vi "VENDING MACHINE.vi"() -> ()   [LabVIEW 2019]
panel:
  out "appended array":T1(array[cluster])
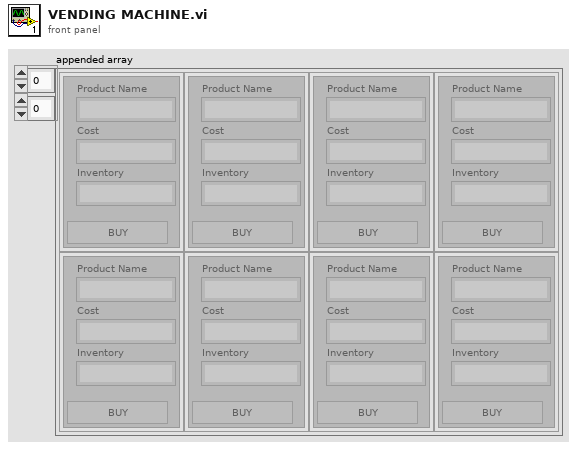
[diagram p1: front panel]
types:
  T1 = cluster{cluster{"Product Name":string, "Cost":string, "Inventory":string, "buy":bool}}[][]
  T2 = cluster{"Product Name":string, "Cost":string, "Inventory":string, "buy":bool}
  T3 = cluster{cluster{"Product Name":string, "Cost":string, "Inventory":string, "buy":bool}}[]
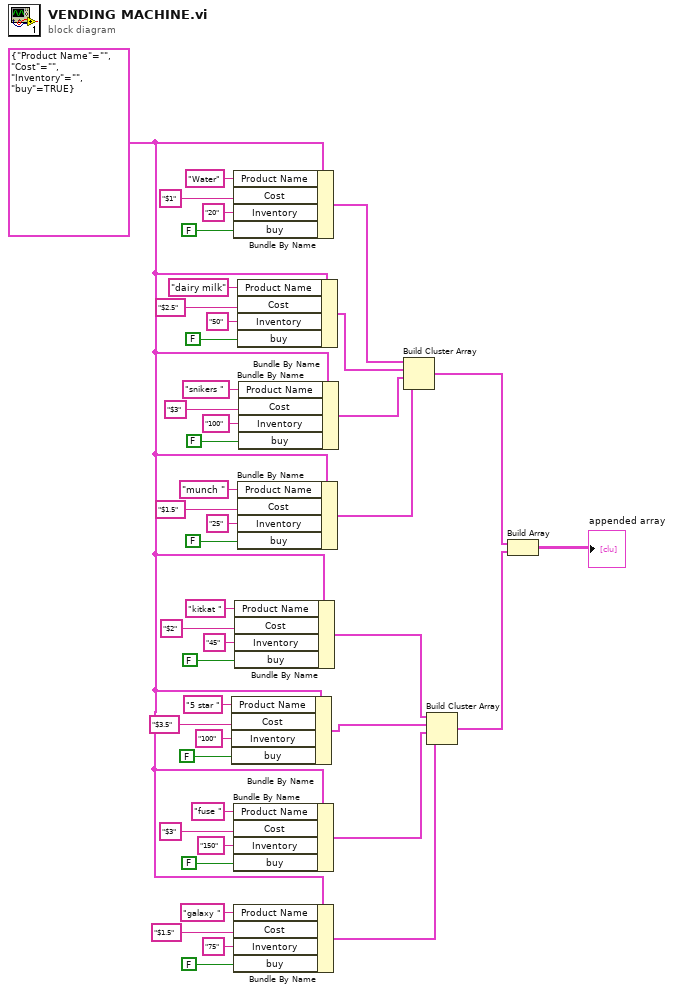
[diagram p0: block diagram]
diagram:
  w7 = T2 {"Product Name"="", "Cost"="", "Inventory"="", "buy"=TRUE}
  n1 = Bundle By Name(cluster=w7, "Product Name"="5 star ", "Cost"="$3.5", "Inventory"="100", "buy"=FALSE) -> (w6:T2)
  n2 = Bundle By Name(cluster=w7, "Product Name"="Water", "Cost"="$1", "Inventory"="20", "buy"=FALSE) -> (w28:T2)
  n3 = Bundle By Name(cluster=w7, "Product Name"="fuse ", "Cost"="$3", "Inventory"="150", "buy"=FALSE) -> (w5:T2)
  n4 = Bundle By Name(cluster=w7, "Product Name"="galaxy ", "Cost"="$1.5", "Inventory"="75", "buy"=FALSE) -> (w4:T2)
  n5 = Bundle By Name(cluster=w7, "Product Name"="kitkat ", "Cost"="$2", "Inventory"="45", "buy"=FALSE) -> (w8:T2)
  n6 = Bundle By Name(cluster=w7, "Product Name"="dairy milk", "Cost"="$2.5", "Inventory"="50", "buy"=FALSE) -> (w27:T2)
  n7 = Bundle By Name(cluster=w7, "Product Name"="munch ", "Cost"="$1.5", "Inventory"="25", "buy"=FALSE) -> (w25:T2)
  n8 = Bundle By Name(cluster=w7, "Product Name"="snikers ", "Cost"="$3", "Inventory"="100", "buy"=FALSE) -> (w26:T2)
  n9 = Build Cluster Array(w28, w27, w26, w25) -> (w3:T3)
  n10 = Build Cluster Array(w8, w6, w5, w4) -> (w2:T3)
  n11 = Build Array(w3, w2) -> (→"appended array":T1)
